vi "GetSystemDefinitionPropertyValue_I32.vi"(8 "error in (no error)":errorcluster, 10 "property name":string, 11 "BaseNodeType in":refnum<k24>) -> (0 "error out":errorcluster, 2 "value":i32, 3 "BaseNodeType out":refnum<k24>)   [LabVIEW 2016, in "VeriStandTestUtilities.lvlib"]
uses:
  VeriStandTestUtilities.lvlib
  NationalInstruments.VeriStand.SystemStorage
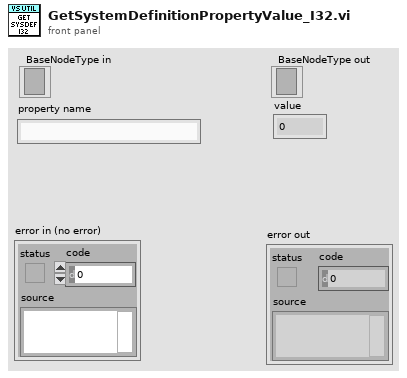
[diagram p1: front panel]
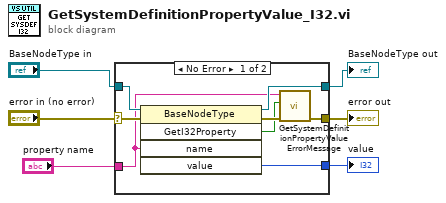
[diagram p0: block diagram]
diagram:
  n1 = case shown="No Error" "error in (no error)" {
    selector: "error in (no error)" -> [w13 w16]
    tunnel: "BaseNodeType in" -> [w14 w15]
    tunnel: "property name" -> [w7 _]
    tunnel: [w12 w15] -> w3
    tunnel: [w9 w16] -> w2
    tunnel: [w11 _] -> w1
    frame No Error {
      n2 = invoke class="BaseNodeType" method="GetI32Property"(reference=w14, error in=w13, "name"=w7) -> (reference out=w12:refnum<k24>, error out=w10:errorcluster, "GetI32Property"=w8:bool, "value"=w11:i32)  [unwired: 2 in, 1 out]
      n3 = call "GetSystemDefinitionPropertyValueErrorMessage.vi"("error in (no error)"=w10, "successful?"=w8, "property name"=w7) -> ("error out"=w9:errorcluster)  [unwired: 8 in]
    }
    frame Error {
    }
  }
  "error out" <- w2
  "BaseNodeType out" <- w3
  "value" <- w1
